vi "Lookup Command.vi"(10 "error in (no error)":refnum<class "MultiErrors.lvclass">, 11 "Command Config":refnum<class "Command Config.lvclass">) -> (2 "error out":refnum<class "MultiErrors.lvclass">, 3 "Command":refnum<class "Command.lvclass">)   [LabVIEW 2020, in "VolatusSeq.lvlib" / "Command.lvclass"]
uses:
  Command.lvclass
  VolatusSeqConfig/Command Config/Command Config.lvclass
  VolatusErrorUtilities/MultiErrors/MultiErrors.lvclass
  Command.lvclass/Command.ctl
  VolatusSeqConfig/Command Type.ctl
  VolatusSeqConfig/VolatusSeqConfig.lvlib
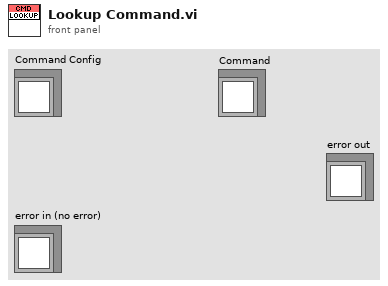
[diagram p1: front panel]
types:
  T1 = typedef "VolatusSeqConfig.lvlib/Command Type.ctl" = enum16{"Digital", "Numeric", "Transition", "Stop", "StartLog", "StopLog"}
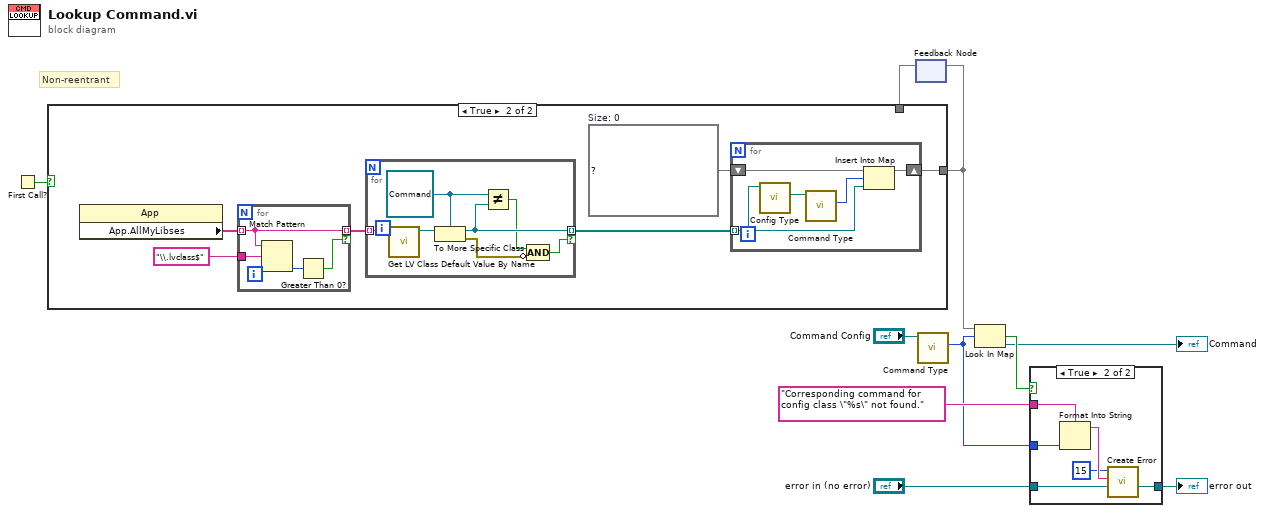
[diagram p0: block diagram]
diagram:
  # "Non-reentrant"
  n1 = First Call?() -> (First Call?: T/F=w10:bool)
  n2 = feedback #1() -> (w8:map{T1, refnum<class "Command.lvclass">})  [unwired: 1 in]
  n3 = case shown="True" w10 {
    tunnel: [w11 w12] -> w7
    tunnel: w8 -> [w11 _]
    frame False {
    }
    frame True {
      w14 = map{T1, refnum<class "Command.lvclass">} {}  # Size: 0
      n4 = property class="App"() -> ("App.AllMyLibses"=w17:string[])  [unwired: 2 in, 2 out]
      n5 = for {
        tunnel: w17 -> [w31] mode=indexing
        tunnel: "\\.lvclass$" -> [w33]
        tunnel: [w31] -> w15 mode=indexing if=w30
        n6 = Match Pattern(string=w31, regular expression=w33) -> (offset past match=w32:i32)  [unwired: 1 in, 3 out]
        n7 = Greater Than 0?(x=w32) -> (x > 0?=w30:bool)
      }
      n8 = for {
        tunnel: w15 -> [w29] mode=indexing
        tunnel: [w26] -> w13 mode=indexing if=w23
        w27 = refnum<class "Command.lvclass"> refnum ("VolatusSeq.lvlib:Command.lvclass")
        n9 = call <vilib>:"Get LV Class Default Value By Name.vi"("class name"=w29) -> ("object"=w28:refnum<class>)  [unwired: 9 in, 1 out]
        n10 = To More Specific Class(target class=w27, reference=w28) -> (specific class reference=w26:refnum<class "Command.lvclass">, error out=w24:errorcluster)  [unwired: 1 in]
        n11 = Not Equal?(x=w27, y=w26) -> (x != y?=w25:bool)
        n12 = Compound Arithmetic op=AND(w25, invert w24) -> (w23:bool)
      }
      n13 = for {
        shift-right: [w21] -> w12
        shift-left: w14 -> [w22]
        tunnel: w13 -> [w20] mode=indexing
        n14 = call-dynamic "Config Type.vi"("Command in"=w20) -> ("Command Config Type"=w19:refnum<class "Command Config.lvclass">)  [unwired: 10 in]
        n15 = call-dynamic "Command Type.vi"("Command Config in"=w19) -> ("Command Type"=w18:T1)  [unwired: 10 in]
        n16 = Insert Into Map(map in=w22, key=w18, value=w20) -> (map out=w21:map{T1, refnum<class "Command.lvclass">})  [unwired: 2 out]
      }
    }
  }
  n17 = feedback-in #1(w7) -> ()
  n18 = call-dynamic "Command Type.vi"("Command Config in"="Command Config") -> ("Command Type"=w4:T1)  [unwired: 10 in]
  n19 = Look In Map(map=w7, key=w4) -> (key not found?=w6:bool, value=→"Command":refnum<class "Command.lvclass">)  [unwired: 1 in]
  n20 = case shown="True" w6 {
    tunnel: "Corresponding command for config class \"%s\" not found." -> [_ w40]
    tunnel: w4 -> [_ w39]
    tunnel: [w34 w36] -> w2
    tunnel: "error in (no error)" -> [w34 w35]
    frame False {
    }
    frame True {
      n21 = Format Into String(format string=w40, w39) -> (resulting string=w38:string)  [unwired: 2 in, 1 out]
      n22 = call "Create Error.vi"("MultiErrors in"=w35, "Message"=w38, "Code"=15 ("error code (0)")) -> ("MultiErrors out"=w36:refnum<class "MultiErrors.lvclass">)  [unwired: 8 in]
    }
  }
  "error out" <- w2
